vi "Capture Single Image.vi"(5 "calRefPath":u8[](array[numeric])=array[4097 elements], 6 "nMode":T1 items=["ACQ_INIT"=0, "DARK_MODE"=1, "BRIGHT_MODE"=2, "SOFTTRIGGER_MODE"=258, "SOFTTRIGGER_INSTANT_MODE"=259], 7 "nWidth":u32, 8 "error in (no error)":errorcluster, 9 "nHeight":u32, 10 "pImage":u16[](array[numeric])=array[4097 elements], 11 "nSensorIP":u32) -> (0 "error out":errorcluster, 2 "pImage out":u16[](array[numeric]), 3 "function return":i32)   [LabVIEW 2017, in "BonTechDetector.lvlib"]
doc: "extern \"C\" BONTECHLIBRARY_API int __stdcall CaptureSingleImage(unsigned int nSensorIP, unsigned short* pImage, unsigned int nHeight, unsigned int nWidth, unsigned int nMode, LPCTSTR calRefPath);"
uses:
  BonTechDetector.lvlib
  Controls/Acquisition Commands.ctl
  BonTechWrapperLibrary.dll
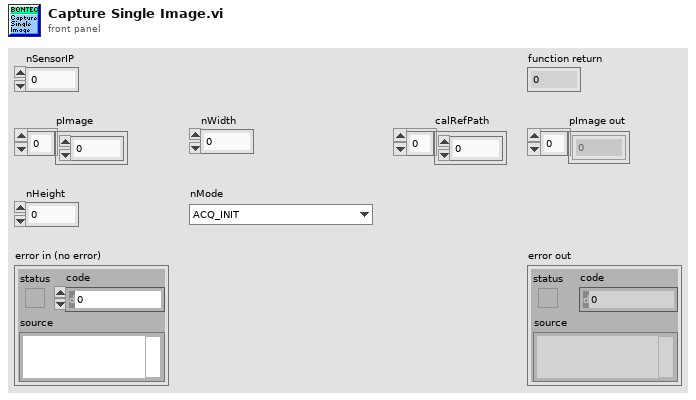
[diagram p1: front panel]
types:
  T1 = typedef "BonTechDetector.lvlib/Acquisition Commands.ctl" = u32
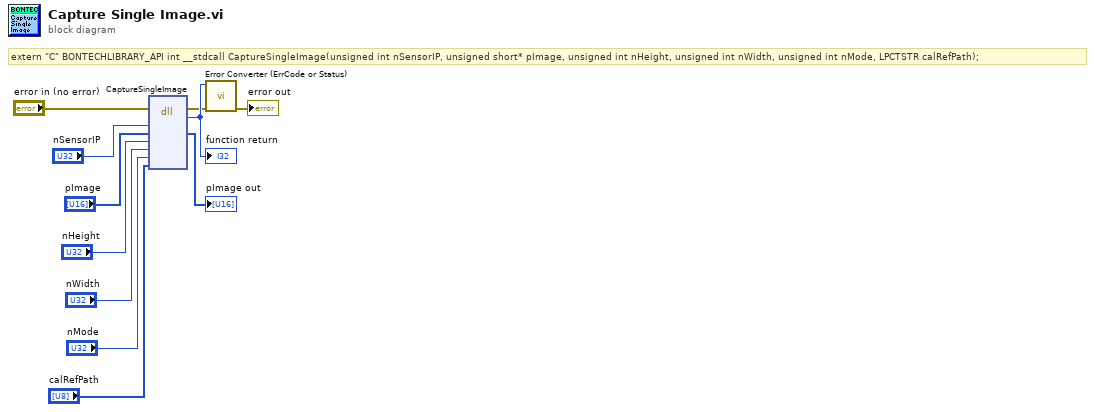
[diagram p0: block diagram]
diagram:
  # "extern \"C\" BONTECHLIBRARY_API int __stdcall CaptureSingleImage(unsigned int nSensorIP, unsigned short* pImage, unsigned int nHeight, unsigned int nWidth, unsigned int nMode, LPCTSTR calRefPath);"
  n1 = dll-call lib="C:/Users/Achuthaperumal/SourceCodes/BonTechFlatPanelLVDriver/LabVIEW Library/BonTechWrapperLibrary.*" fn="CaptureSingleImage"(error in="error in (no error)", "nSensorIP"="nSensorIP", "pImage"="pImage", "nHeight"="nHeight", "nWidth"="nWidth", "nMode"="nMode", "calRefPath"="calRefPath") -> (error out=w2:errorcluster, w11:i32, "pImage"=→"pImage out":u16[])  [unwired: 7 in, 1 out]
  "function return" <- w11
  n2 = call "Error Converter (ErrCode or Status).vi"("error in (no error)"=w2, "error code"=w11) -> ("error out"=→"error out":errorcluster)  [unwired: 9 in]
